vi "State_Machine.vi"(8 "error in (no error)":errorcluster caption="entrée d'erreur (pas d'erreur)", 11 "Get_Voltage en entrée":refnum<class "Open_Instr.lvclass">) -> (0 "error out":errorcluster caption="sortie d'erreur", 2 "Json_String":string, 3 "Get_Voltage en sortie":refnum<class "Open_Instr.lvclass">)   [LabVIEW 2020, in "Library Test.lvlib" / "Open_Instr.lvclass"]
uses:
  Open_Instr.lvclass
  C:/Users/ngarcin/OneDrive - Altyor/Standard TB/Suite TB45/Class/Test/Test (Default)/Test (Default).lvclass
  Commun VI/TypeDef/Variable Printable.ctl
  Instrument/Instrument (Default)/Class Instrument (Default).lvclass
  Commun VI/Library Commun.lvlib
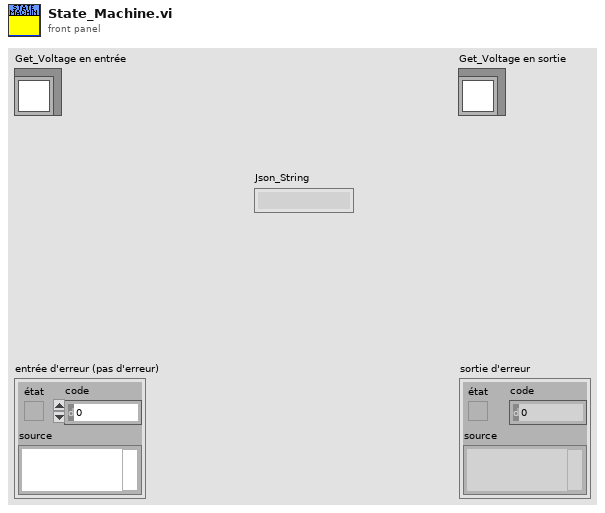
[diagram p1: front panel]
types:
  T1 = typedef "Variable Printable.ctl" = string
  T2 = enum16{"Get Variable", "Get All Variables", "Set Variable", "Delete Variable", "Delete All Variable"}
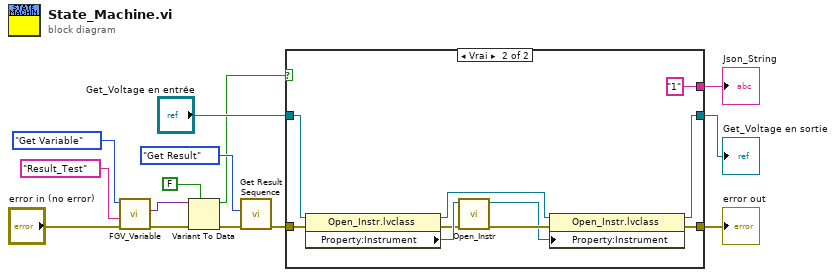
[diagram p0: block diagram]
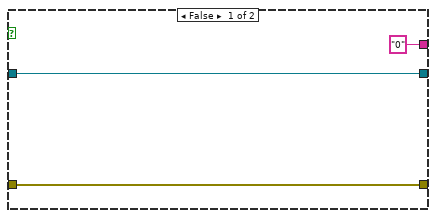
[diagram p2: hidden frame]
diagram:
  n1 = call "FGV_Variable.vi"("error in (no error)"="error in (no error)", "Variable"=T1 "Result_Test", "Function"=T2."Get Variable") -> ("error out"=w6:errorcluster, "Data Out"=w5:variant)  [unwired: 6 in, 1 out]
  n2 = Variant To Data(error in=w6, type=FALSE, Variant=w5) -> (data=w1:bool, error out=w2:errorcluster)
  n3 = call "Get Result Sequence.vi"("error in (no error)"=w2, "Function"=enum16{"Get Result", "Reset", "Set Result"}."Get Result") -> ("error out"=w11:errorcluster)  [unwired: 8 in, 1 out]
  n4 = case shown="Vrai" w1 {
    tunnel: "Get_Voltage en entrée" -> [w17 w27]
    tunnel: [w16 w20] -> w13
    tunnel: [w17 w21] -> w12
    tunnel: w11 -> [w16 w26]
    tunnel: ["0" "1"] -> w9
    frame False {
    }
    frame True {
      n5 = property class="Open_Instr.lvclass"(reference=w27, error in=w26) -> (reference out=w22:refnum<class "Open_Instr.lvclass">, error out=w23:errorcluster, "Property:Instrument"=w24:refnum<class "Class Instrument (Default).lvclass">)
      n6 = call-dynamic "Open_Instr.vi"("error in (no error)"=w23, "Class Multimeter (Default) en entrée"=w24) -> ("error out"=w19:errorcluster, "Class Multimeter (Default) en sortie"=w18:refnum<class "Class Instrument (Default).lvclass">)  [unwired: 8 in]
      n7 = property class="Open_Instr.lvclass"(reference=w22, error in=w19, "Property:Instrument"=w18) -> (reference out=w21:refnum<class "Open_Instr.lvclass">, error out=w20:errorcluster)
    }
  }
  "error out" <- w13
  "Get_Voltage en sortie" <- w12
  "Json_String" <- w9
